vi "ARTIQ-Client Delete Command.vi"(8 "error in (no error)":errorcluster, 11 "Kasli Wrapper 2.0 in":refnum<class "Kasli Wrapper 2.0.lvclass">) -> (0 "error out":errorcluster, 2 "artiq-client delete":string, 3 "Kasli Wrapper 2.0 out":refnum<class "Kasli Wrapper 2.0.lvclass">)   [LabVIEW 2020, in "Kasli Wrapper 2.0.lvlib" / "Kasli Wrapper 2.0.lvclass"]
uses:
  Kasli Wrapper 2.0.lvclass
  Kasli Wrapper 2.0.lvclass/Kasli Wrapper 2.0.ctl
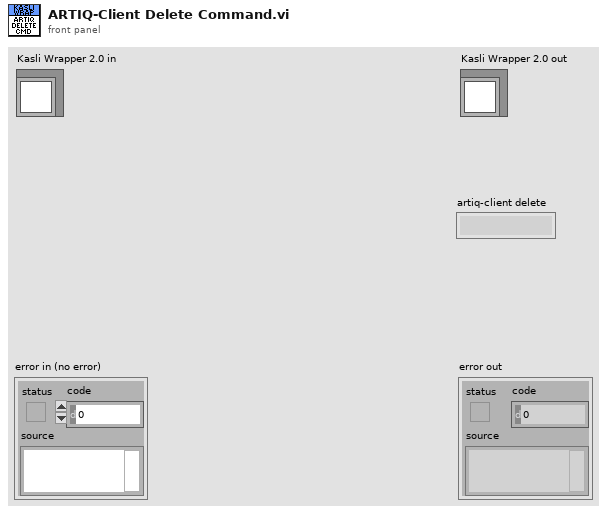
[diagram p1: front panel]
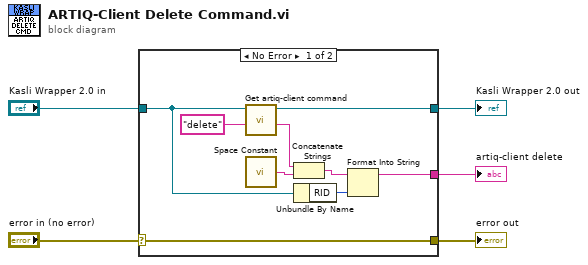
[diagram p0: block diagram]
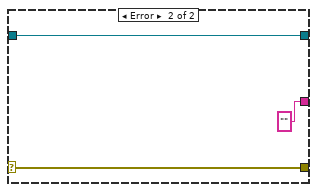
[diagram p2: hidden frame]
diagram:
  n1 = case shown="No Error" "error in (no error)" {
    selector: "error in (no error)" -> [w14 w17]
    tunnel: [w14 w17] -> w4
    tunnel: [w12 w16] -> w2
    tunnel: "Kasli Wrapper 2.0 in" -> [w9 w16]
    tunnel: [w6 ""] -> w1
    frame No Error {
      n2 = call-dynamic "Get artiq-client command.vi"("sub-command"="delete" ("string"), "Kasli Wrapper 2.0 in"=w9) -> ("command"=w10:string, "Kasli Wrapper 2.0 out"=w12:refnum<class "Kasli Wrapper 2.0.lvclass">)  [unwired: 8 in]
      n3 = call <vilib>:"Space Constant.vi"() -> ("String"=w11:string)
      n4 = Concatenate Strings(w10, w11) -> (w7:string)
      n5 = Unbundle By Name(w9) -> ("RID"=w8:u32)
      n6 = Format Into String(initial string=w7, w8) -> (resulting string=w6:string)  [unwired: 2 in, 1 out]
    }
    frame Error {
    }
  }
  "error out" <- w4
  "Kasli Wrapper 2.0 out" <- w2
  "artiq-client delete" <- w1
